vi "Save Matrix.vi"(4 "section":string, 5 "Matrix 2":dbl[][](array[numeric]), 6 "error in (no error)":errorcluster, 7 "Matrix 1":dbl[][](array[numeric]), 8 "Keys":string[](array[string]), 9 "refnum in":T2) -> (0 "error out":errorcluster, 2 "refnum out":T2)   [LabVIEW 2013]
uses:
  <vilib>/Utility/config.llb/Config Data RefNum.ctl
  Metadata/LBCB Number.ctl
  <vilib>/Utility/config.llb/Write Key (String).vi
  <vilib>/Utility/config.llb/NI_LVConfig.lvlib
panel:
  in  "LBCB Number":T1
  in  "delimiter":string="."
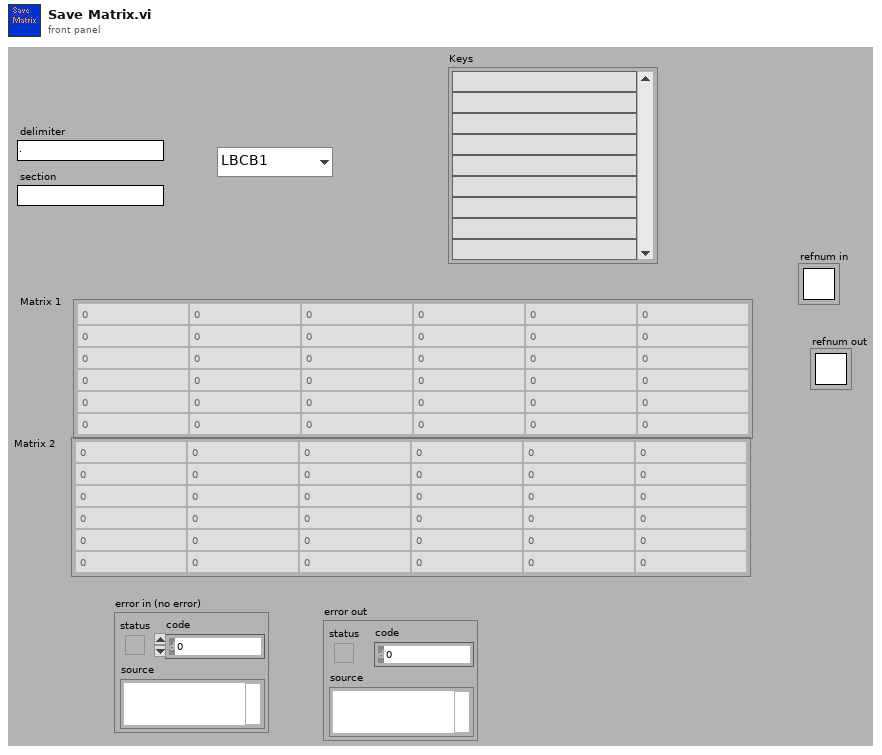
[diagram p1: front panel]
types:
  T1 = typedef "LBCB Number.ctl" = enum16{"LBCB1", "LBCB2"}
  T2 = typedef "NI_LVConfig.lvlib/Config Data RefNum.ctl" = refnum<k1>
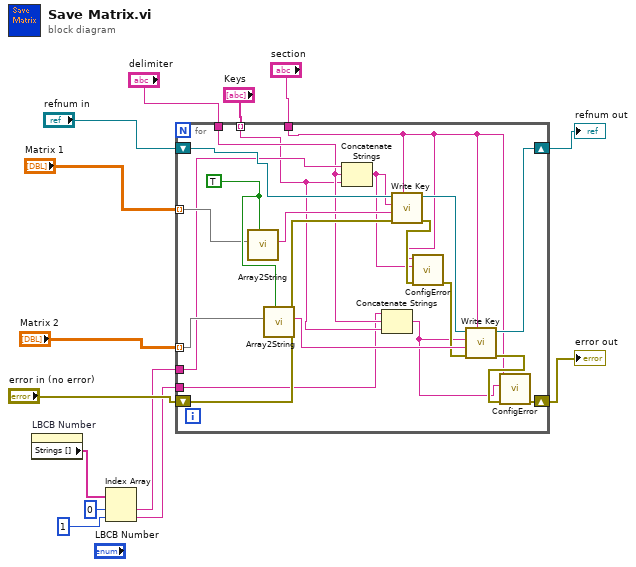
[diagram p0: block diagram]
diagram:
  n1 = property on="LBCB Number" class="Enum (strict)"() -> ("Strings []"=w3:string[])  [unwired: 2 in, 2 out]
  n2 = Index Array(array=w3, index #1=0 ("index"), index #2=1 ("index")) -> (element #1=w2:string, element #2=w1:string)
  n3 = for {
    tunnel: w2 -> [w19]
    tunnel: w1 -> [w16]
    shift-right: [w33] -> w7
    shift-left: "refnum in" -> [w34]
    shift-right: [w22] -> w9
    shift-left: "error in (no error)" -> [w32]
    tunnel: "section" -> [w20]
    tunnel: "Keys" -> [w17] mode=indexing
    tunnel: "Matrix 2" -> [w27] mode=indexing
    tunnel: "Matrix 1" -> [w29] mode=indexing
    tunnel: "delimiter" -> [w18]
    w30 = TRUE ("Use Space")
    n4 = call "Array2String.vi"("Use Space"=w30, "Array"=w29) -> ("String"=w28:string)  [unwired: 9 out]
    n5 = call "Array2String.vi"("Use Space"=w30, "Array"=w27) -> ("String"=w26:string)  [unwired: 9 out]
    n6 = Concatenate Strings(w19, w18, w17) -> (w21:string)
    n7 = Concatenate Strings(w16, w18, w17) -> (w15:string)
    n8 = call-poly <vilib>:"Write Key.vi"("section"=w20, "error in (no error)"=w32, "value"=w28, "key"=w21, "refnum"=w34) -> ("error out"=w25:errorcluster, "refnum out"=w31:T2)  [unwired: 1 in, 4 out]
    n9 = call "ConfigError.vi"("error in (no error)"=w25, "Key"=w21, "Section"=w20) -> ("error out"=w24:errorcluster)  [unwired: 8 out]
    n10 = call-poly <vilib>:"Write Key.vi"("section"=w20, "error in (no error)"=w24, "value"=w26, "key"=w15, "refnum"=w31) -> ("error out"=w23:errorcluster, "refnum out"=w33:T2)  [unwired: 1 in, 4 out]
    n11 = call "ConfigError.vi"("error in (no error)"=w23, "Key"=w15, "Section"=w20) -> ("error out"=w22:errorcluster)  [unwired: 8 out]
  }
  "error out" <- w9
  "refnum out" <- w7
